vi "BRig_dataTrial_I_listeningRig.vi"() -> (2 "output_I_listeningRig":i32)   [LabVIEW 2014]
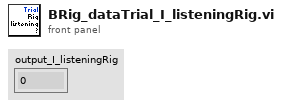
[diagram p1: front panel]
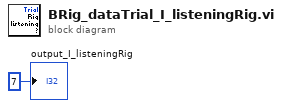
[diagram p0: block diagram]
diagram:
  "output_I_listeningRig" <- 7 ("output_iBlock")
